vi "Read Coords.vi"(8 "error in (no error)":errorcluster, 11 "ControlMouseUpMsg in":refnum<class "ControlMouseUpMsg.lvclass">) -> (0 "error out":errorcluster, 2 "Coords":T1, 3 "ControlMouseUpMsg out":refnum<class "ControlMouseUpMsg.lvclass">)   [LabVIEW 2017, in "ActorEvents.lvlib" / "ControlMouseUpMsg.lvclass"]
uses:
  ControlMouseUpMsg.lvclass
  <vilib>/Utility/miscctls.llb/LVPoint32TypeDef.ctl
  ControlMouseUpMsg.lvclass/ControlMouseUpMsg.ctl
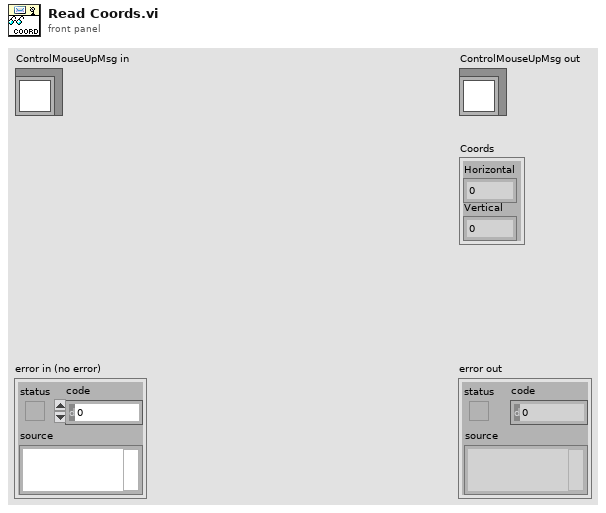
[diagram p1: front panel]
types:
  T1 = typedef "LVPoint32TypeDef.ctl" = cluster{"Horizontal":i32, "Vertical":i32}
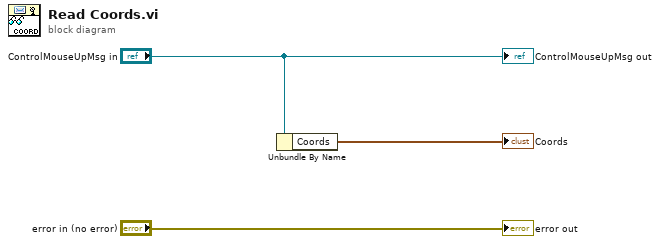
[diagram p0: block diagram]
diagram:
  n1 = Unbundle By Name("ControlMouseUpMsg in") -> ("Coords"=→"Coords":T1)
  "error out" <- "error in (no error)"
  "ControlMouseUpMsg out" <- "ControlMouseUpMsg in"
